vi "Fpga-Uart-State-Machine.vi"() -> ()   [LabVIEW 2017]
uses:
  <vilib>/Platform/TimedLoop/XDataNode/timing_clust.ctl
  <vilib>/Platform/TimedLoop/XDataNode/nitl_modes.ctl
  <vilib>/Platform/TimedLoop/XDataNode/wakeup.ctl
  UART.States.ctl
  UART.States.2.ctl
  <vilib>/rvi/Emulation/niFpgaSctlEmulationGetInTimedLoop.vi
  <vilib>/rvi/Emulation/niFpgaEmulationReportErrorSimple.vi
  <vilib>/rvi/Emulation/niFpgaGetClockAttributes.vi
  <vilib>/rvi/Emulation/niFpgaCriticalErrorInLSC.vi
  <vilib>/rvi/eio/common/nirviEmuTemplateMethod_errors.vi
  <vilib>/rvi/interface/RandomDataEmulation/niFpgaRandomDataHandleErrors.vi
  <vilib>/Platform/TimedLoop/XDataNode/XDataNode.xnode
  <vilib>/eio/EIONode/EIONode.xnode
  <vilib>/rvi/DataTransferAndStorage/Container/XNode/niFpgaContainer.xnode
  <vilib>/rvi/interface/RandomDataEmulation/nirviRandomDataFpgaReadWriteTemplate.vi
  <vilib>/Platform/TimedLoop/XDataNode/XDNodeRunTimeDep.lvlib
panel:
  out "Half Bit":u32
  out "Full Bit":u32
  in  "gpio_rtl_tri_i":u32
  out "gpio_rtl_0_tri_o":u32
  in  "uart_rtl_rxd":bool=TRUE
  in  "reset_rtl":bool
  in  "Baud Rate":u32(ring)=128000 items=["110"=110, "300"=300, "1200"=1200, "2400"=2400, "4800"=4800, "9600"=9600, "19200"=19200, "38400"=38400, "57600"=57600, "115200"=115200, "128000"=128000, "230400"=230400, "460800"=460800, "921600"=921600]
  in  "FPGA Clock Rate (MHz)":u32=100
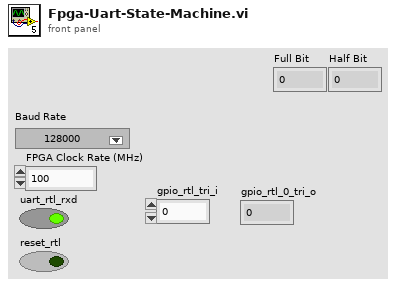
[diagram p1: front panel]
types:
  T1 = typedef "UART.States.2.ctl" = enum16{"No-Wait", "Wait-Half", "Wait-Full", "Wait-One-and-a-Half"}
  T2 = typedef "UART.States.ctl" = enum16{"Read-StartBit", "Read-DataBits", "Read-Parity", "Read-StopBit", "Shift"}
  T3 = typedef "XDNodeRunTimeDep.lvlib/timing_clust.ctl" = cluster{"Expected End [f-1]":u64, "Actual End [f-1]":u64, "Finished Late? [f-1]":bool, "Expected End [i-1]":u64, "Actual End [i-1]":u64, "Finished Late? [i-1]":bool, "Expected Start [i]":u64, "Actual Start [i]":u64, "Expected Start [f]":u64, "Actual Start [f]":u64, "Source Name":string, "Structure Name":string, "Period":i64, "Deadline":i64, "Offset":i64, "Start":i64, "Priority":i32, "Timeout":i32, "Mode":T4, "Wakeup Reason":T5, "Error":errorcluster, "Source Type":string, "Secondary Source Type":string, "Global End Time":u64, "Global Start Time":u64, "Frame Duration":u64, "Iteration Duration":u64, "Assigned CPU":i32, "I/O Scan Engine Mode":u32}
  T4 = typedef "XDNodeRunTimeDep.lvlib/nitl_modes.ctl" = enum32{"No Change", "Process missed periods, maintain original phase", "Discard missed periods, maintain original phase", "Process missed periods, ignore original phase", "Discard missed periods, ignore original phase"}
  T5 = typedef "XDNodeRunTimeDep.lvlib/wakeup.ctl" = enum32{"Normal", "Aborted", "Asynchronous wakeup", "Timing source error", "Timed loop error", "Timeout"}
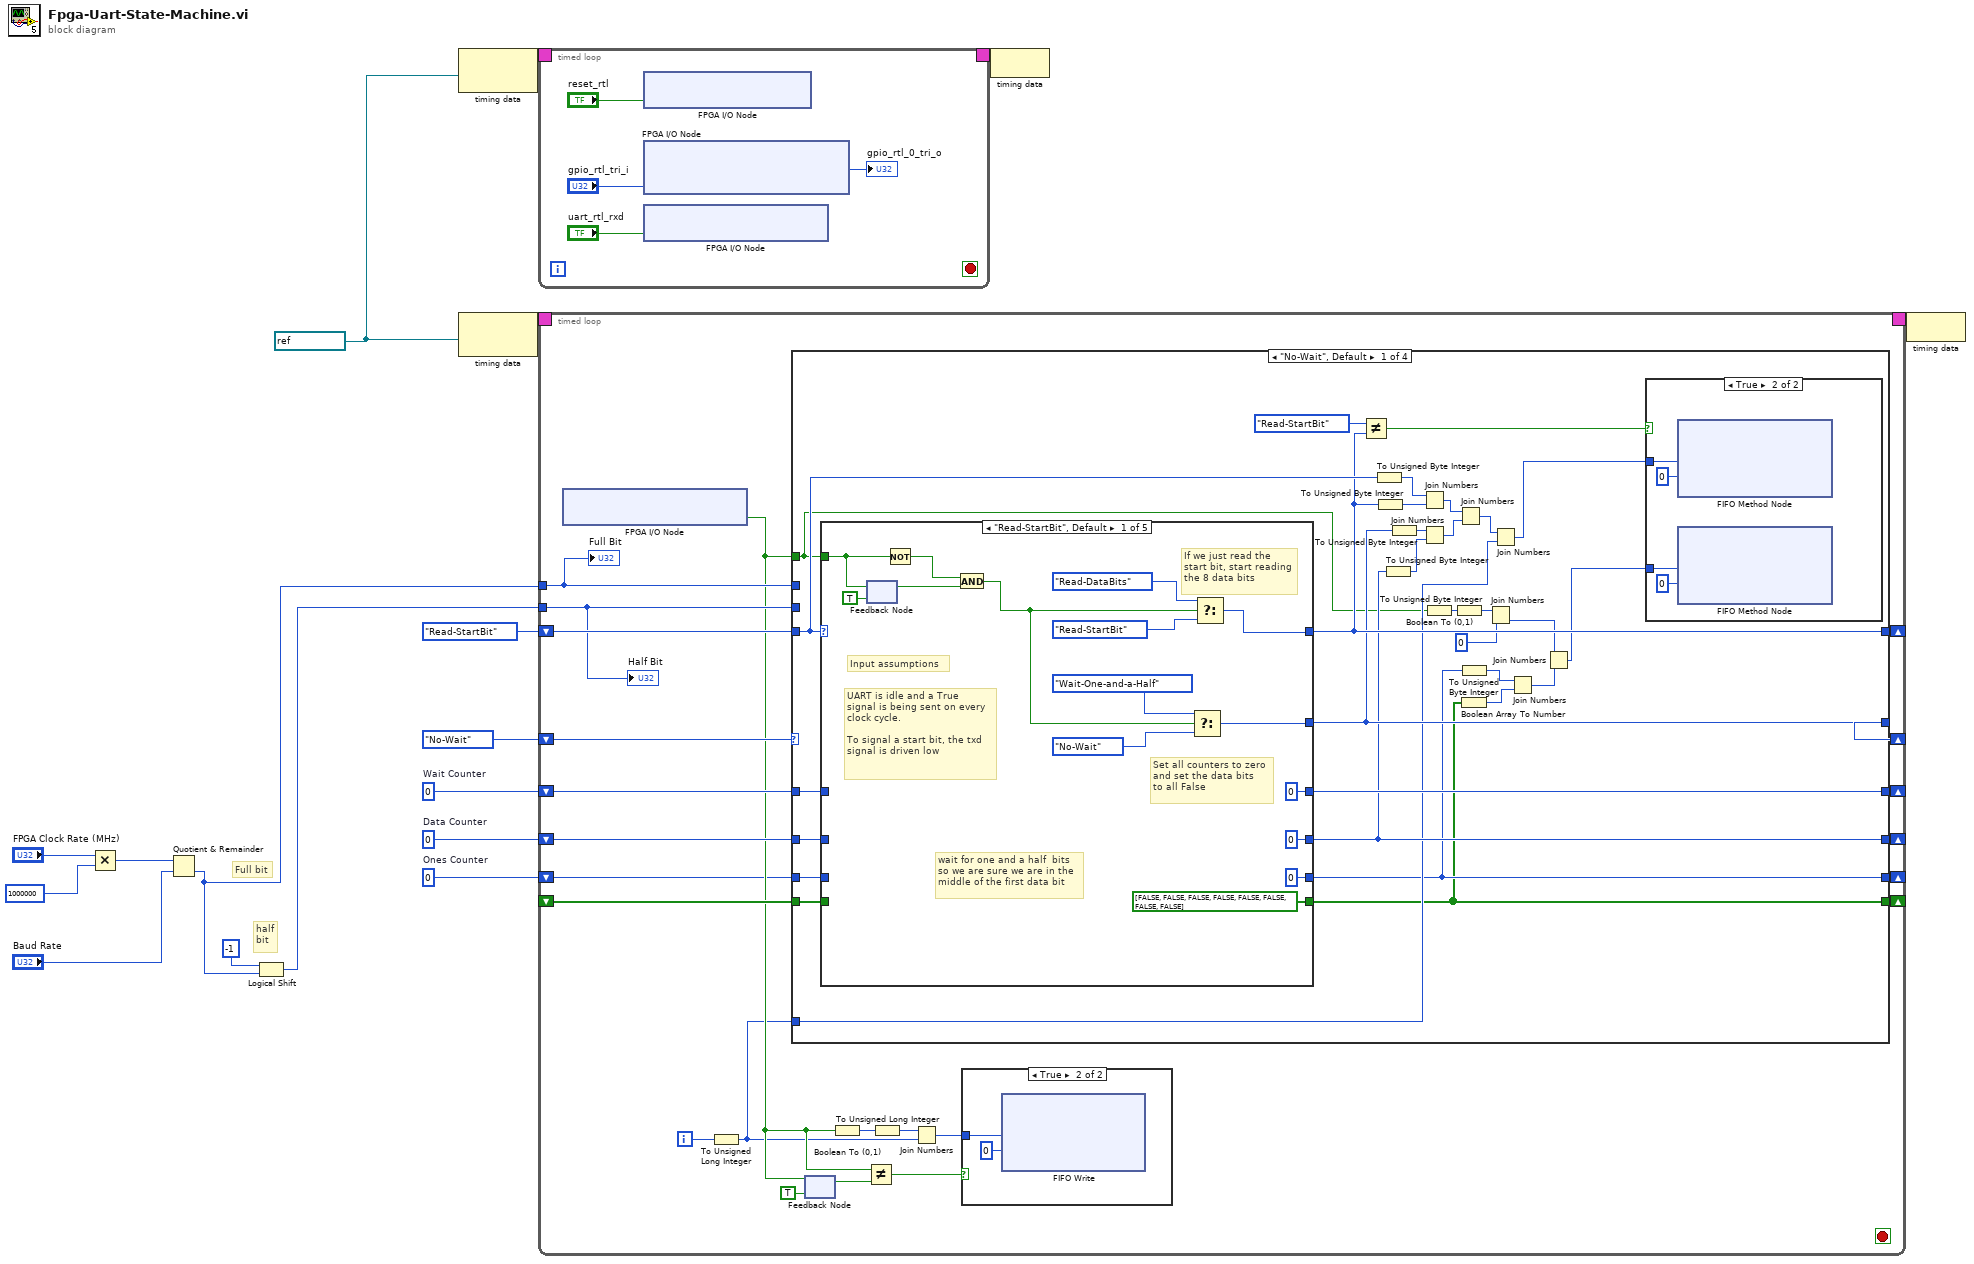
[diagram p0: block diagram]
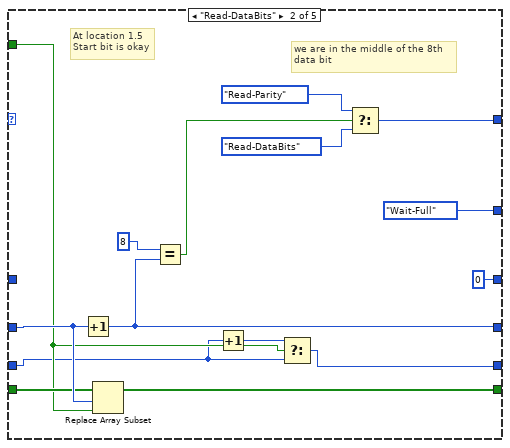
[diagram p4: hidden frame]
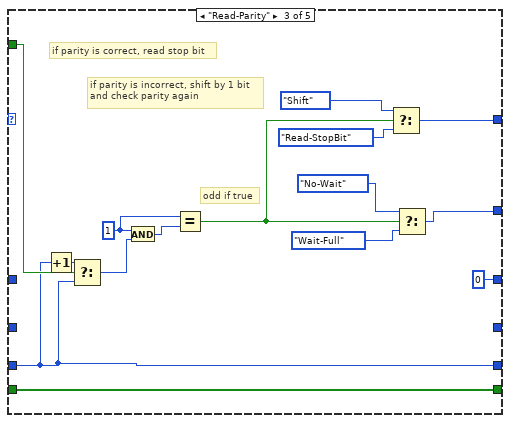
[diagram p5: hidden frame]
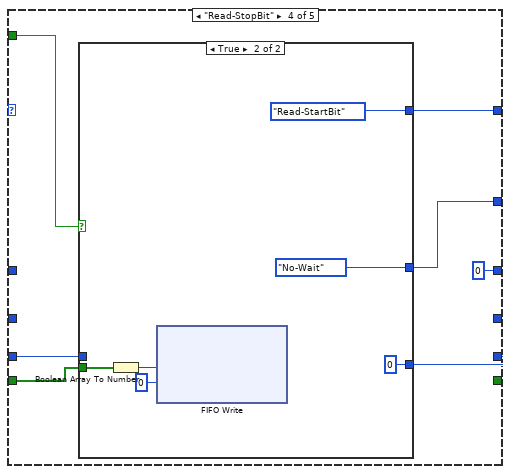
[diagram p6: hidden frame]
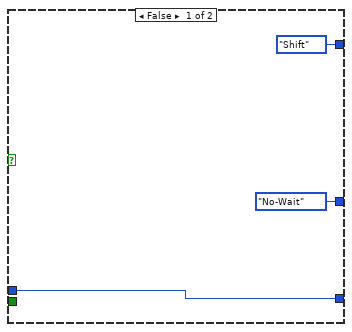
[diagram p7: hidden frame]
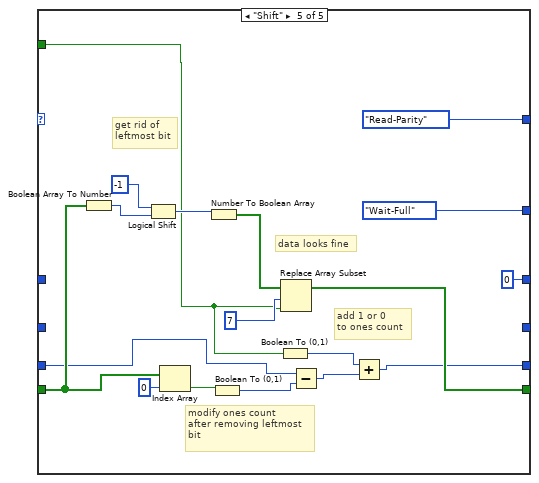
[diagram p8: hidden frame]
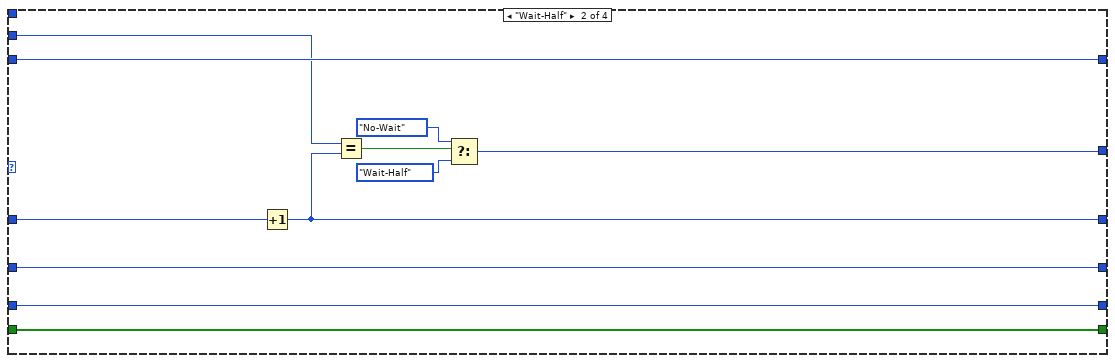
[diagram p9: hidden frame]
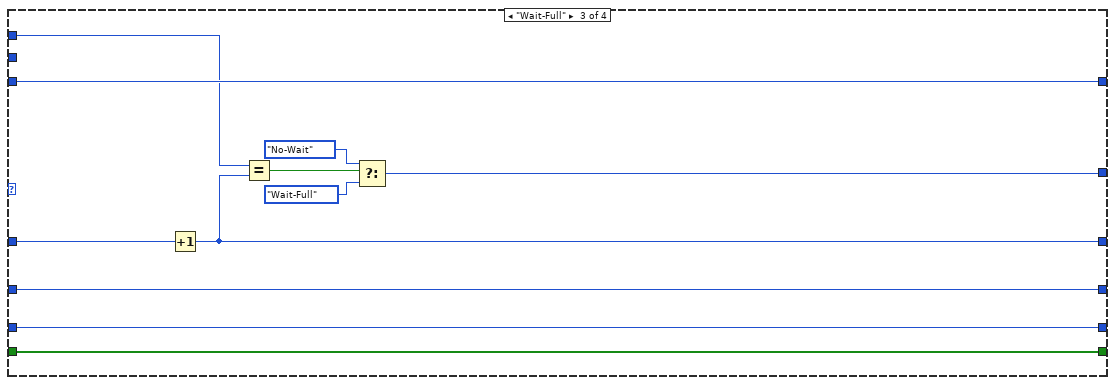
[diagram p10: hidden frame]
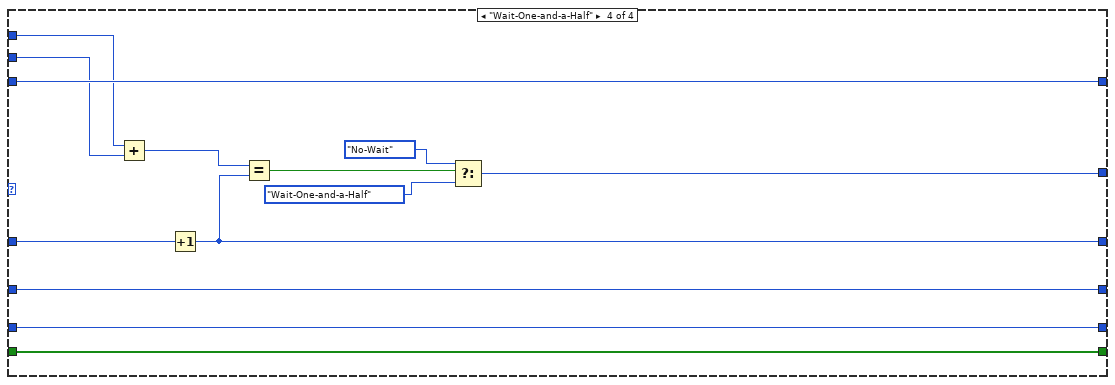
[diagram p11: hidden frame]
diagram:
  w1 = u32 0  # Ones Counter
  w5 = u32 0  # Data Counter
  w6 = u32 0  # Wait Counter
  w9 = refnum<k21> "100MHz" ("Source Name")
  # "half\nbit"
  # "Full bit"
  n1 = Multiply(x="FPGA Clock Rate (MHz)", y=u32 1000000) -> (x*y=w16:u32)
  n2 = Quotient & Remainder(x=w16, y="Baud Rate") -> (floor(x/y)=w2:u32)  [unwired: 1 out]
  n3 = Logical Shift(y=i16 -1, x=w2) -> (x << y=w3:u32)
  n4 = node-c288(w9) -> (w13:T3)
  n5 = node-c288(w9) -> (w11:T3)
  n6 = timed-loop {
    timing: w13 -> [_]
    timing-out: [_] -> w12
    stop <- _ stop-if-true
    n7 = xnode "FPGA I/O Node"("d_microblaze_i\\reset_rtl"="reset_rtl") -> ()  [unwired: 1 in, 1 out]
    n8 = xnode "FPGA I/O Node"("d_microblaze_i\\gpio_rtl_tri_i"="gpio_rtl_tri_i") -> ("d_microblaze_i\\gpio_rtl_0_tri_o"=→"gpio_rtl_0_tri_o":u32)  [unwired: 2 in, 2 out]
    n9 = xnode "FPGA I/O Node"("d_microblaze_i\\uart_rtl_rxd"="uart_rtl_rxd") -> ()  [unwired: 1 in, 1 out]
  }
  n10 = timed-loop {
    timing: w11 -> [_]
    timing-out: [_] -> w10
    shift-right: [w45] -> _
    shift-left: UART.States."Read-StartBit" -> [w46]
    shift-right: [w43] -> _
    shift-left: UART.States.2."No-Wait" -> [w44]
    shift-right: [w40] -> _
    shift-left: w6 -> [w42]
    shift-right: [w39] -> _
    shift-left: w5 -> [w41]
    tunnel: w2 -> [w38]
    tunnel: w3 -> [w37]
    shift-right: [w36] -> _
    shift-left: _ -> [w35]
    shift-right: [w25] -> _
    shift-left: w1 -> [w26]
    i -> [w29]
    stop <- _ stop-if-true
    n11 = xnode "FPGA I/O Node"() -> ("d_microblaze_i\\uart_rtl_txd"=w30:bool)  [unwired: 1 in, 1 out]
    n12 = To Unsigned Long Integer(number=w29) -> (unsigned 32bit integer=w24:u32)
    n13 = case shown="\"No-Wait\", Default" w44 {
      tunnel: w46 -> [w73 w167 w176 w189]
      tunnel: w30 -> [w55 _ _ _]
      tunnel: [w72 w167 w176 w189] -> w45
      tunnel: [w69 w168 w180 w193] -> w43
      tunnel: w42 -> [w79 w173 w181 w194]
      tunnel: w41 -> [w78 w166 w179 w192]
      tunnel: [w67 w172 w178 w191] -> w40
      tunnel: [w65 w166 w179 w192] -> w39
      tunnel: w38 -> [_ _ w175 w187]
      tunnel: w37 -> [_ w164 _ w186]
      tunnel: [w57 w165 w177 w190] -> w36
      tunnel: w35 -> [w77 w165 w177 w190]
      tunnel: w26 -> [w76 w163 w174 w188]
      tunnel: [w59 w163 w174 w188] -> w25
      tunnel: w24 -> [w61 _ _ _]
      frame "No-Wait", Default {
        n14 = case shown="\"Read-StartBit\", Default" w73 {
          tunnel: w55 -> [w95 w103 w128 w134 w149]
          tunnel: [w94 w104 w124 w132 UART.States."Read-Parity"] -> w72
          tunnel: [w88 UART.States.2."Wait-Full" w119 w133 UART.States.2."Wait-Full"] -> w69
          tunnel: w79 -> [_ _ _ _ _]
          tunnel: w78 -> [_ w112 _ _ _]
          tunnel: [u32 0 ("Wait Counter") u32 0 ("Wait Counter") u32 0 ("Wait Counter") u32 0 ("Wait Counter") u32 0 ("Wait Counter")] -> w67
          tunnel: [u32 0 ("Data Counter") w109 _ _ _] -> w65
          tunnel: [bool[] [FALSE, FALSE, FALSE, FALSE, FALSE, FALSE, FALSE, FALSE] w110 w117 _ w155] -> w57
          tunnel: w77 -> [_ w111 w117 w135 w154]
          tunnel: w76 -> [_ w102 w115 w130 w152]
          tunnel: [u32 0 ("Data Counter") w100 w115 w131 w147] -> w59
          frame "Read-StartBit", Default {
            # "Set all counters to zero\nand set the data bits\nto all False"
            # "wait for one and a half  bits\nso we are sure we are in the\nmiddle of the first data bit"
            # "If we just read the \nstart bit, start reading\nthe 8 data bits"
            # "UART is idle and a True\nsignal is being sent on every\nclock cycle.\n\nTo signal a start bit, the txd\nsignal is driven low"
            # "Input assumptions"
            n15 = feedback #1(TRUE ("d_microblaze_i\\uart_rtl_txd")) -> (w98:bool)
            n16 = feedback-in #1(w95) -> ()
            n17 = Not(x=w95) -> (.not. x?=w97:bool)
            n18 = And(x=w97, y=w98) -> (x .and. y?=w91:bool)
            n19 = Select(t=UART.States.2."Wait-One-and-a-Half", s=w91, f=UART.States.2."No-Wait") -> (s? t:f=w88:T1)
            n20 = Select(t=UART.States."Read-DataBits", s=w91, f=UART.States."Read-StartBit") -> (s? t:f=w94:T2)
          }
          frame "Read-DataBits" {
            # "we are in the middle of the 8th\ndata bit"
            # "At location 1.5\nStart bit is okay"
            n21 = Increment(x=w112) -> (x+1=w109:u32)
            n22 = Replace Array Subset(array=w111, new element=w103, index=w112) -> (w110:bool[])
            n23 = Equal?(x=u32 8, y=w109) -> (x = y?=w107:bool)
            n24 = Increment(x=w102) -> (x+1=w101:u32)
            n25 = Select(t=w101, s=w103, f=w102) -> (s? t:f=w100:u32)
            n26 = Select(t=UART.States."Read-Parity", s=w107, f=UART.States."Read-DataBits") -> (s? t:f=w104:T2)
          }
          frame "Read-Parity" {
            w125 = u32 1 ("x")
            # "odd if true"
            # "if parity is incorrect, shift by 1 bit\nand check parity again"
            # "if parity is correct, read stop bit"
            n27 = Increment(x=w115) -> (x+1=w127:u32)
            n28 = Select(t=w127, s=w128, f=w115) -> (s? t:f=w116:u32)
            n29 = And(x=w125, y=w116) -> (x .and. y?=w126:u32)
            n30 = Equal?(x=w125, y=w126) -> (x = y?=w121:bool)
            n31 = Select(t=UART.States."Shift", s=w121, f=UART.States."Read-StopBit") -> (s? t:f=w124:T2)
            n32 = Select(t=UART.States.2."No-Wait", s=w121, f=UART.States.2."Wait-Full") -> (s? t:f=w119:T1)
          }
          frame "Read-StopBit" {
            n33 = case shown="True" w134 {
              tunnel: w135 -> [_ w142]
              tunnel: [UART.States.2."No-Wait" UART.States.2."No-Wait"] -> w133
              tunnel: [UART.States."Shift" UART.States."Read-StartBit"] -> w132
              tunnel: [w136 u32 0 ("Ones Counter")] -> w131
              tunnel: w130 -> [w136 _]
              frame False {
              }
              frame True {
                n34 = Boolean Array To Number(Boolean array=w142) -> (number=w144:u8)
                n35 = xnode ("FIFO Write")("Element"=w144, "Timeout"=0) -> ()  [unwired: 1 in, 2 out]
              }
            }
          }
          frame "Shift" {
            # "data looks fine"
            # "add 1 or 0\nto ones count"
            # "modify ones count\nafter removing leftmost\nbit"
            # "get rid of\nleftmost bit"
            n36 = Boolean Array To Number(Boolean array=w154) -> (number=w162:u8)
            n37 = Logical Shift(y=i16 -1, x=w162) -> (x << y=w160:u8)
            n38 = Index Array(array=w154, index=0) -> (element=w153:bool)
            n39 = Number To Boolean Array(number=w160) -> (Boolean array=w157:bool[])
            n40 = Boolean To (0,1)(Boolean=w153) -> (0, 1=w151:i16)
            n41 = Boolean To (0,1)(Boolean=w149) -> (0, 1=w148:i16)
            n42 = Replace Array Subset(array=w157, new element=w149, index=7) -> (w155:bool[])
            n43 = Subtract(x=w152, y=w151) -> (x-y=w150:u32)
            n44 = Add(x=w148, y=w150) -> (x+y=w147:u32)
          }
        }
        n45 = Not Equal?(x=UART.States."Read-StartBit", y=w72) -> (x != y?=w74:bool)
        n46 = To Unsigned Byte Integer(number=w73) -> (unsigned 8bit integer=w71:u8)
        n47 = To Unsigned Byte Integer(number=w72) -> (unsigned 8bit integer=w70:u8)
        n48 = To Unsigned Byte Integer(number=w65) -> (unsigned 8bit integer=w66:u8)
        n49 = To Unsigned Byte Integer(number=w69) -> (unsigned 8bit integer=w68:u8)
        n50 = Join Numbers(hi=w71, lo=w70) -> ((hi.lo)=w64:u16)
        n51 = Join Numbers(hi=w68, lo=w66) -> ((hi.lo)=w63:u16)
        n52 = Boolean To (0,1)(Boolean=w55) -> (0, 1=w54:i16)
        n53 = To Unsigned Byte Integer(number=w54) -> (unsigned 8bit integer=w50:u8)
        n54 = Join Numbers(hi=w64, lo=w63) -> ((hi.lo)=w62:u32)
        n55 = To Unsigned Byte Integer(number=w59) -> (unsigned 8bit integer=w58:u8)
        n56 = Boolean Array To Number(Boolean array=w57) -> (number=w56:u8)
        n57 = Join Numbers(hi=w50, lo=u8 0) -> ((hi.lo)=w53:u16)
        n58 = Join Numbers(hi=w62, lo=w61) -> ((hi.lo)=w60:u64)
        n59 = Join Numbers(hi=w58, lo=w56) -> ((hi.lo)=w51:u16)
        n60 = Join Numbers(hi=w53, lo=w51) -> ((hi.lo)=w52:u32)
        n61 = case shown="True" w74 {
          tunnel: w60 -> [_ w81]
          tunnel: w52 -> [_ w80]
          frame False {
          }
          frame True {
            n62 = xnode ("FIFO Method Node")("Element"=w81, "Timeout"=0) -> ()  [unwired: 1 in, 2 out]
            n63 = xnode ("FIFO Method Node")("Element"=w80, "Timeout"=0) -> ()  [unwired: 1 in, 2 out]
          }
        }
      }
      frame "Wait-Half" {
        n64 = Increment(x=w173) -> (x+1=w172:u32)
        n65 = Equal?(x=w164, y=w172) -> (x = y?=w171:bool)
        n66 = Select(t=UART.States.2."No-Wait", s=w171, f=UART.States.2."Wait-Half") -> (s? t:f=w168:T1)
      }
      frame "Wait-Full" {
        n67 = Increment(x=w181) -> (x+1=w178:u32)
        n68 = Equal?(x=w175, y=w178) -> (x = y?=w184:bool)
        n69 = Select(t=UART.States.2."No-Wait", s=w184, f=UART.States.2."Wait-Full") -> (s? t:f=w180:T1)
      }
      frame "Wait-One-and-a-Half" {
        n70 = Add(x=w187, y=w186) -> (x+y=w185:u32)
        n71 = Increment(x=w194) -> (x+1=w191:u32)
        n72 = Equal?(x=w185, y=w191) -> (x = y?=w197:bool)
        n73 = Select(t=UART.States.2."No-Wait", s=w197, f=UART.States.2."Wait-One-and-a-Half") -> (s? t:f=w193:T1)
      }
    }
    n74 = feedback-in #2(w30) -> ()
    n75 = feedback #2(TRUE ("d_microblaze_i\\uart_rtl_txd")) -> (w34:bool)
    n76 = Boolean To (0,1)(Boolean=w30) -> (0, 1=w32:i16)
    n77 = Not Equal?(x=w30, y=w34) -> (x != y?=w33:bool)
    n78 = To Unsigned Long Integer(number=w32) -> (unsigned 32bit integer=w27:u32)
    n79 = Join Numbers(hi=w27, lo=w24) -> ((hi.lo)=w31:u64)
    n80 = case shown="True" w33 {
      tunnel: w31 -> [_ w47]
      frame False {
      }
      frame True {
        n81 = xnode ("FIFO Write")("Element"=w47, "Timeout"=0) -> ()  [unwired: 1 in, 2 out]
      }
    }
    "Full Bit" <- w38
    "Half Bit" <- w37
  }
  n82 = node-c288(w12) -> ()
  n83 = node-c288(w10) -> ()
